vi "CRYMake Asio Buffer.vi"(8 "Fs":u32, 9 "Buffer Index":u32, 10 "Duration(s)":dbl min=0.0 max=1000.0 step=1.0 format="%#.3p", 11 "Data Array":sgl[](array[numeric])) -> (1 "BufferIsEmpty?":bool, 3 "Buf Data":sgl[](array[numeric]))   [LabVIEW 2013]
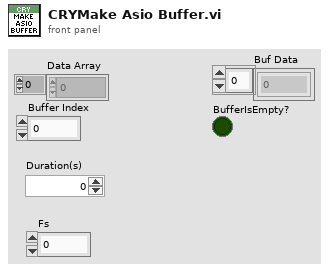
[diagram p1: front panel]
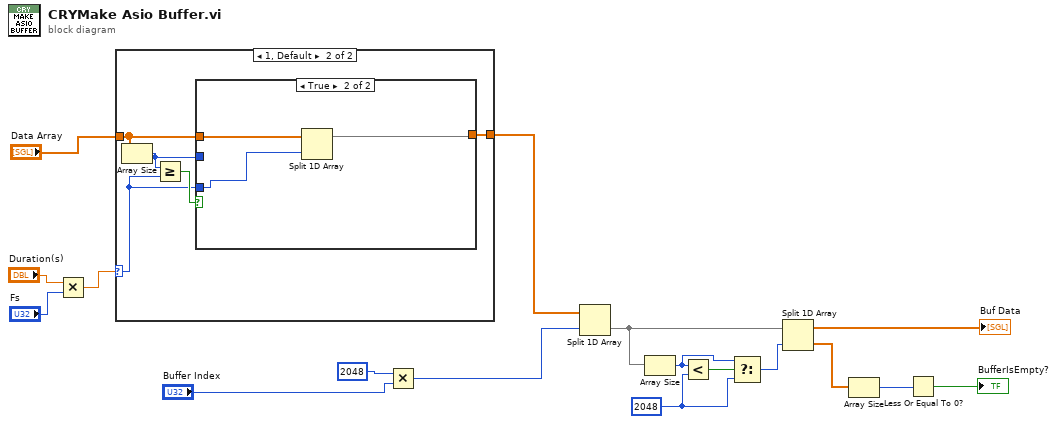
[diagram p0: block diagram]
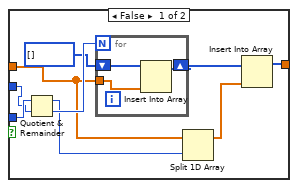
[diagram p3: hidden frame]
diagram:
  w11 = 2048 ("index")
  n1 = Multiply(x="Duration(s)", y="Fs") -> (x*y=w3:dbl)
  n2 = case shown="1, Default" w3 {
    selector: w3 -> [_ w21]
    tunnel: "Data Array" -> [w18 w19]
    tunnel: [w18 w20] -> w1
    frame 0 {
    }
    frame 1, Default {
      n3 = Array Size(array=w19) -> (size(s)=w22:i32)
      n4 = Greater Or Equal?(x=w22, y=w21) -> (x >= y?=w23:bool)
      n5 = case shown="True" w23 {
        tunnel: w22 -> [w31 _]
        tunnel: w21 -> [w32 w36]
        tunnel: w19 -> [w27 w38]
        tunnel: [w24 w37] -> w20
        frame False {
          n6 = Quotient & Remainder(x=w32, y=w31) -> (x-y*floor(x/y)=w26:i32, floor(x/y)=w30:i32)
          n7 = for {
            N: w30 -> [_]
            tunnel: w27 -> [w35]
            shift-right: [w34] -> w28
            shift-left: i32[] [] -> [w33]
            n8 = Insert Into Array(array=w33, new element=w35) -> (w34:i32[])  [unwired: 1 in]
          }
          n9 = Split 1D Array(array=w27, index=w26) -> (first subarray=w25:sgl[])  [unwired: 1 out]
          n10 = Insert Into Array(array=w28, new element=w25) -> (w24:i32[])  [unwired: 1 in]
        }
        frame True {
          n11 = Split 1D Array(array=w38, index=w36) -> (first subarray=w37:sgl[])  [unwired: 1 out]
        }
      }
    }
  }
  n12 = Multiply(x=u32 2048, y="Buffer Index") -> (x*y=w16:u32)
  n13 = Split 1D Array(array=w1, index=w16) -> (second subarray=w14:sgl[])  [unwired: 1 out]
  n14 = Array Size(array=w14) -> (size(s)=w12:i32)
  n15 = Less?(x=w12, y=w11) -> (x < y?=w13:bool)
  n16 = Select(t=w12, s=w13, f=w11) -> (s? t:f=w10:i32)
  n17 = Split 1D Array(array=w14, index=w10) -> (first subarray=→"Buf Data":sgl[], second subarray=w9:sgl[])
  n18 = Array Size(array=w9) -> (size(s)=w8:i32)
  n19 = Less Or Equal To 0?(x=w8) -> (x <= 0?=→"BufferIsEmpty?":bool)
